vi "PSDEV_Device Init Data Queue.vi"(8 "error in":errorcluster caption="错误输入（无错误）", 10 "DeviceIndex":i32, 11 "Card":T1={"Module Type"="", "Module Name"="", "ModuSN"="", "ModuIP"="", "Used?"=FALSE, "Connected"=FALSE, "Timing*"={"Sample Rate"=1000.0}, "Channels"=[]}) -> (0 "error out":errorcluster, 2 "#UsedChannels":i32, 3 "Q Name":string)   [LabVIEW 2016]
uses:
  DAQ-Config/Controls/PSCHN_Channel Para.ctl
  DAQ-Config/Controls/PSCHN_Card Para.ctl
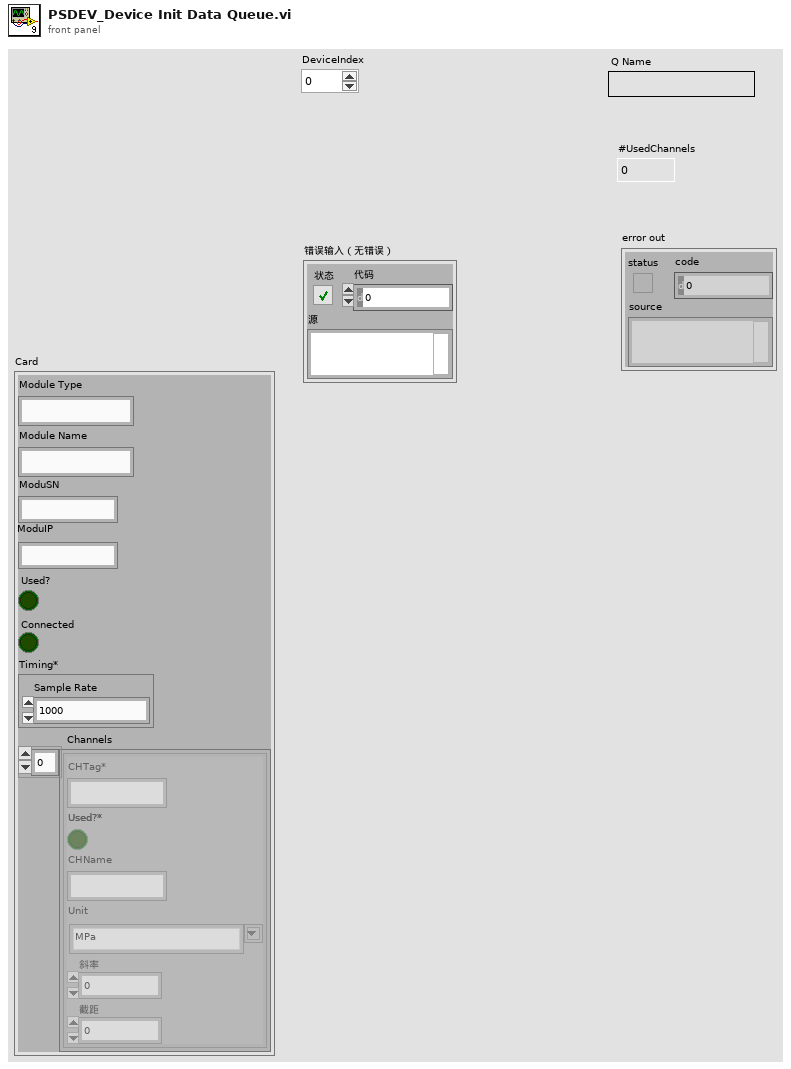
[diagram p1: front panel]
types:
  T1 = typedef "PSCHN_Card Para.ctl" = cluster{"Module Type":string, "Module Name":string, "ModuSN":string, "ModuIP":string, "Used?":bool, "Connected":bool, "Timing*":cluster{"Sample Rate":dbl}, "Channels":T2[]}
  T2 = typedef "PSCHN_Channel Para.ctl" = cluster{"CHTag*":string, "Used?*":bool, "CHName":string, "Unit":string, "斜率":dbl, "截距":dbl}
  T3 = cluster{"Module Name":string, string[], "Object Name":string}
  T4 = cluster{"Queue Name":string, "DAQ Channels":string[], "Queue Type":string}[]
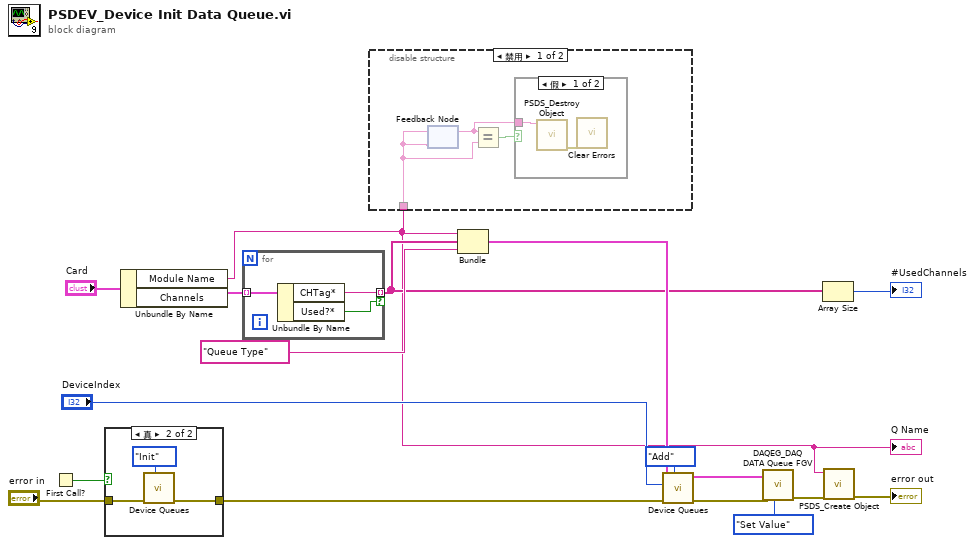
[diagram p0: block diagram]
diagram:
  n1 = First Call?() -> (First Call?: T/F=w8:bool)
  n2 = case shown="真" w8 {
    tunnel: [w18 w20] -> w7
    tunnel: "error in" -> [w18 w19]
    frame False {
    }
    frame True {
      n3 = call "Device Queues.vi"("枚举"=enum16{"Init", "Add", "Read"}."Init", "error in (no error)"=w19) -> ("error out"=w20:errorcluster)  [unwired: 8 in, 1 out]
    }
  }
  n4 = Unbundle By Name("Card") -> ("Module Name"=w2:string, "Channels"=w16:T2[])
  "Q Name" <- w2
  n5 = for {
    tunnel: w16 -> [w24] mode=indexing
    tunnel: [w23] -> w3 mode=indexing if=w22
    n6 = Unbundle By Name(w24) -> ("CHTag*"=w23:string, "Used?*"=w22:bool)
  }
  n7 = disable-structure shown="禁用" {
    disable-tunnel: w2 -> [w25 _]
    frame Disabled {
      n8 = feedback #1(w25) -> (w26:string)
      n9 = feedback-in #1(w25) -> ()
      n10 = Equal?(x=w26, y=w25) -> (x = y?=w27:bool)
      n11 = case shown="假" w27 {
        tunnel: w26 -> [w29 _]
        frame False {
          n12 = call "PSDS_Destroy Object.vi"("Object Name"=w29) -> ("error out"=w28:errorcluster)  [unwired: 10 in]
          n13 = call <vilib>:"Clear Errors.vi"("error in (no error)"=w28) -> ()  [unwired: 5 in, 2 out]
        }
        frame True {
        }
      }
    }
    frame Enabled {
    }
  }
  n14 = Bundle("Module Name"=w2, w3, "Object Name"="Queue Type") -> (w11:T3)  [unwired: 1 in]
  n15 = call "Device Queues.vi"("枚举"=enum16{"Init", "Add", "Read"}."Add", "error in (no error)"=w7, "DeviceIndex"="DeviceIndex", "DAQ Data"=w11) -> ("error out"=w6:errorcluster, "DAQ Data[] out"=w12:T4)  [unwired: 6 in]
  n16 = call "DAQEG_DAQ DATA Queue FGV.vi"("Command"=enum16{"Initialize", "Get Value", "Set Value"}."Set Value", "error in (no error)"=w6, "DAQ DATA"=w12) -> ("error out"=w14:errorcluster)  [unwired: 7 in, 1 out]
  n17 = Array Size(array=w3) -> (size(s)=→"#UsedChannels":i32)
  n18 = call "PSDS_Create Object.vi"("error in (no error)"=w14, "Object Name"=w2) -> ("error out"=→"error out":errorcluster)  [unwired: 8 in, 1 out]
